vi "create rtd data directory v3.vi"(4 "error in":errorcluster, 6 "Base path":path=path "C:/Users/LAB319D/gitHIPPOS", 7 "description":string) -> (0 "error out":errorcluster, 3 "dir path":path)   [LabVIEW 2018]
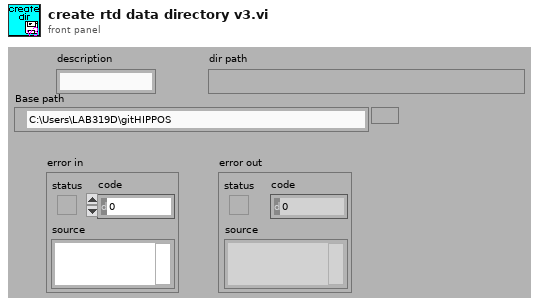
[diagram p1: front panel]
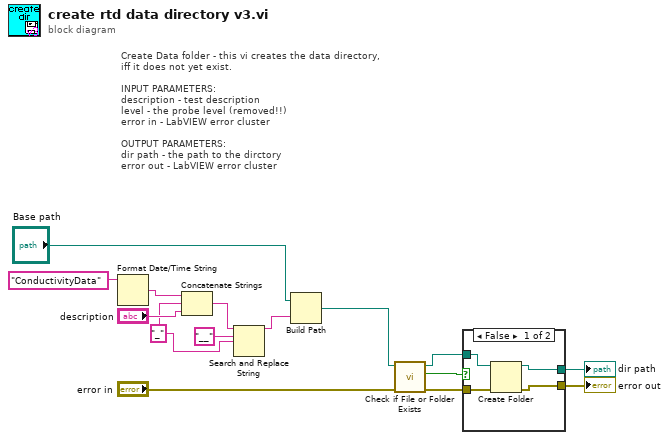
[diagram p0: block diagram]
diagram:
  w1 = "_" ("replace string (\"\")")
  # "Create Data folder - this vi creates the data directory,\niff it does not yet exist.\n\nINPUT PARAMETERS:\ndescription - test description\nlevel - the probe level (removed!!)\nerror in - LabVIEW error cluster\n\nOUTPUT PARAMETERS:\ndir path - the path to the dirctory\nerror out - LabVIEW error cluster"
  n1 = Format Date/Time String(time format string (%c)="ConductivityData") -> (date/time string=w13:string)  [unwired: 2 in]
  n2 = Concatenate Strings(w13, w1, "description") -> (w5:string)
  n3 = Search and Replace String(input string=w5, search string="__", replace string=w1) -> (result string=w4:string)  [unwired: 5 in, 3 out]
  n4 = Build Path(base path="Base path", name or relative path=w4) -> (appended path=w8:path)
  n5 = call <vilib>:"Check if File or Folder Exists.vi"("error in (no error)"="error in", "path"=w8) -> ("error out"=w10:errorcluster, "file or folder exists?"=w12:bool, "dup path"=w7:path)  [unwired: 7 in]
  n6 = case shown="False" w12 {
    tunnel: w10 -> [w19 w21]
    tunnel: w7 -> [w18 w20]
    tunnel: [w17 w20] -> w6
    tunnel: [w16 w21] -> w9
    frame False {
      n7 = Create Folder(path (use dialog)=w18, error in=w19) -> (created path=w17:path, error out=w16:errorcluster)  [unwired: 1 in, 1 out]
    }
    frame True {
    }
  }
  "error out" <- w9
  "dir path" <- w6
